vi "Verificador_leitura_de_forma.vi"() -> ()   [LabVIEW 2017]
uses:
  <vilib>/userdefined/High Color/IMAQdx.ctl
  <vilib>/vision/driver/IMAQdx.llb/IMAQdx Acquisition Mode.ctl
  <vilib>/vision/driver/IMAQdx.llb/IMAQdx Buffer Number Mode.ctl
  <vilib>/vision/Classification.llb/IMAQ Classifier Read Options.ctl
  <vilib>/vision/driver/NI_Vision_Acquisition_Software.lvlib
  <vilib>/vision/NI_Vision_Development_Module.lvlib
panel:
  out "Forma 2":string
  out "Imagem Original 2":T1(plugin-control)
  out "Session Out":T2
  out "error out":errorcluster
  out "Forma":string
  out "Points":cluster{"X":dbl, "Y":dbl}[](array[cluster])
  in  "error in":errorcluster
  out "Stop 3":bool
  out "lista":enum16{"normal", "detectou", "parou"}(ring)=enum."detectou"
  in  "enum":enum16{"normal", "detectou", "parou"}(ring)=enum."detectou"
  in  "Stop Button":bool
  in  "largura_y":sgl=30.0
  in  "largura_x":sgl=30.0
  in  "ofset y":sgl
  in  "ofset x":sgl
  in  "Tab Control":T3(tab)
  in  "Stop 2":bool
  in  "Stop 1":bool
  out "Imagem Original":T1(plugin-control)
  in  "Câmera":T2="cam1"
  # "0"
  # "-250"
  # "400"
  # "80"
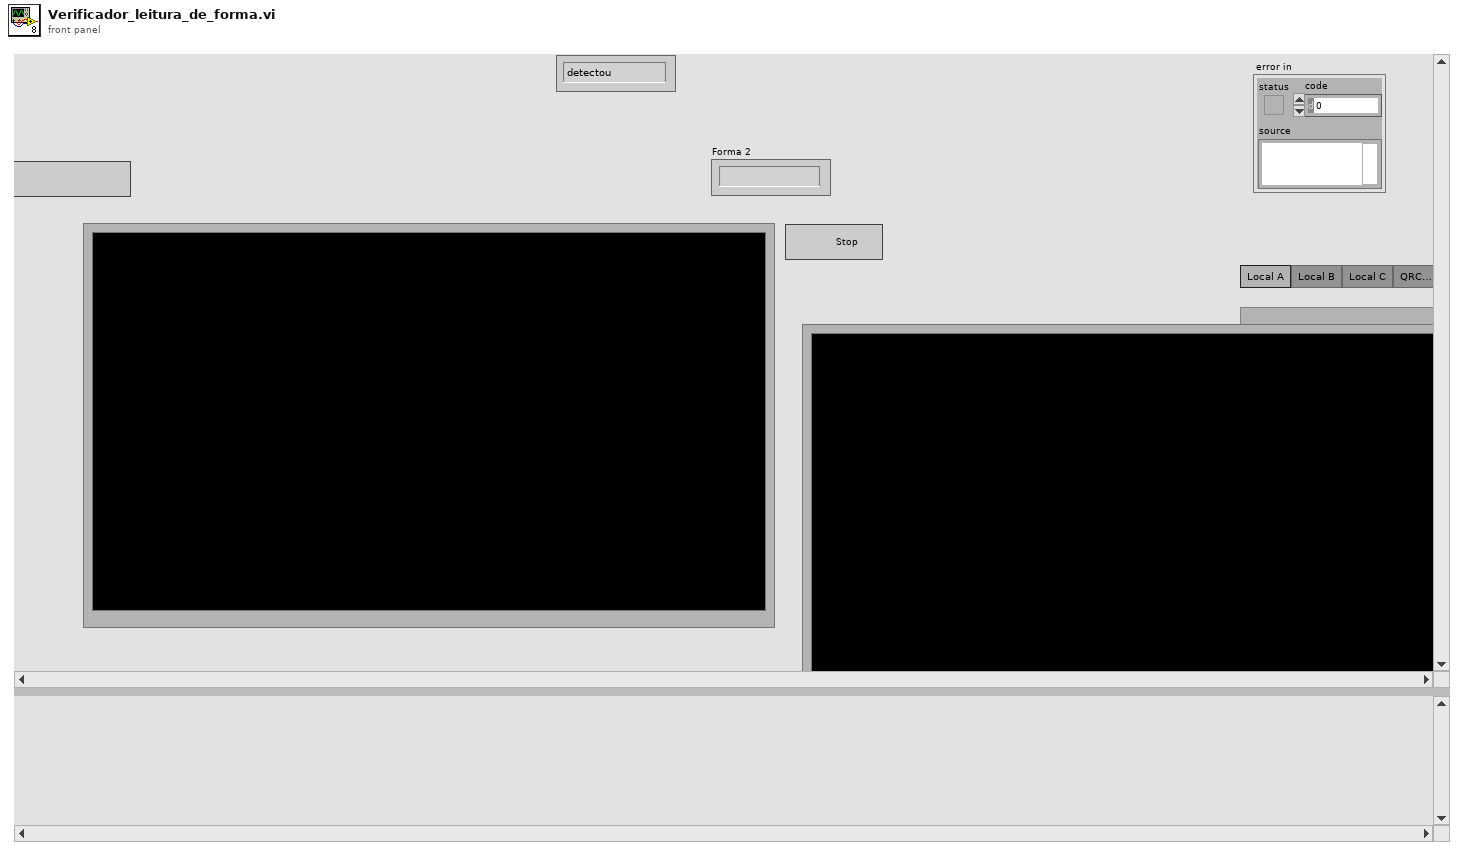
[diagram p1: front panel]
types:
  T1 = typedef "IMAQ Image.ctl" = refnum<image>
  T2 = typedef "IMAQdx.ctl" = refnum<k21>
  T3 = enum32{"Local A", "Local B", "Local C", "QRCode"}
  T4 = typedef "NI_Vision_Acquisition_Software.lvlib/IMAQdx Acquisition Mode.ctl" = enum32{"One Shot", "Continuous"}
  T5 = typedef "NI_Vision_Acquisition_Software.lvlib/IMAQdx Buffer Number Mode.ctl" = enum32{"Next", "Last", "Buffer Number", "Every", "Last New"}
  T6 = cluster{"Global Rectangle":i32[], "Contours":cluster{"Contour Type":u32, "ROI Type":u32, "Points":i32[]}[]}
  T7 = enum32{"AutoM", "Close", "Dilate", "Erode", "Gradient", "Gradient out", "Gradient in", "Hit miss", "Open", "PClose", "POpen", "Thick", "Thin"}
  T8 = typedef "ROI Descriptor" = cluster{"Global Rectangle":i32[], "Contours":cluster{"ID":enum32{"External", "Internal"}, "Type":u32, "Coordinates":i32[]}[]}
  T9 = typedef "IMAQ Classifier Read Options.ctl" = i32
  T10 = typedef "IMAQ Classifier Session.ctl" = refnum<k1>
  T11 = cluster{"Contour Type":u32, "ROI Type":u32, "Points":i32[]}[]
  T12 = cluster{"Contour Type":u32, "ROI Type":u32, "Points":i32[]}
  T13 = typedef "Image Type" = u32
  T14 = typedef "IMAQ ExtractCurvesCurve.ctl" = cluster{"Points":cluster{"X":dbl, "Y":dbl}[], "Closed?":bool, "Curve Length":dbl, "Min Edge Strength":dbl, "Max Edge Strength":dbl, "Average Edge Strength":dbl}
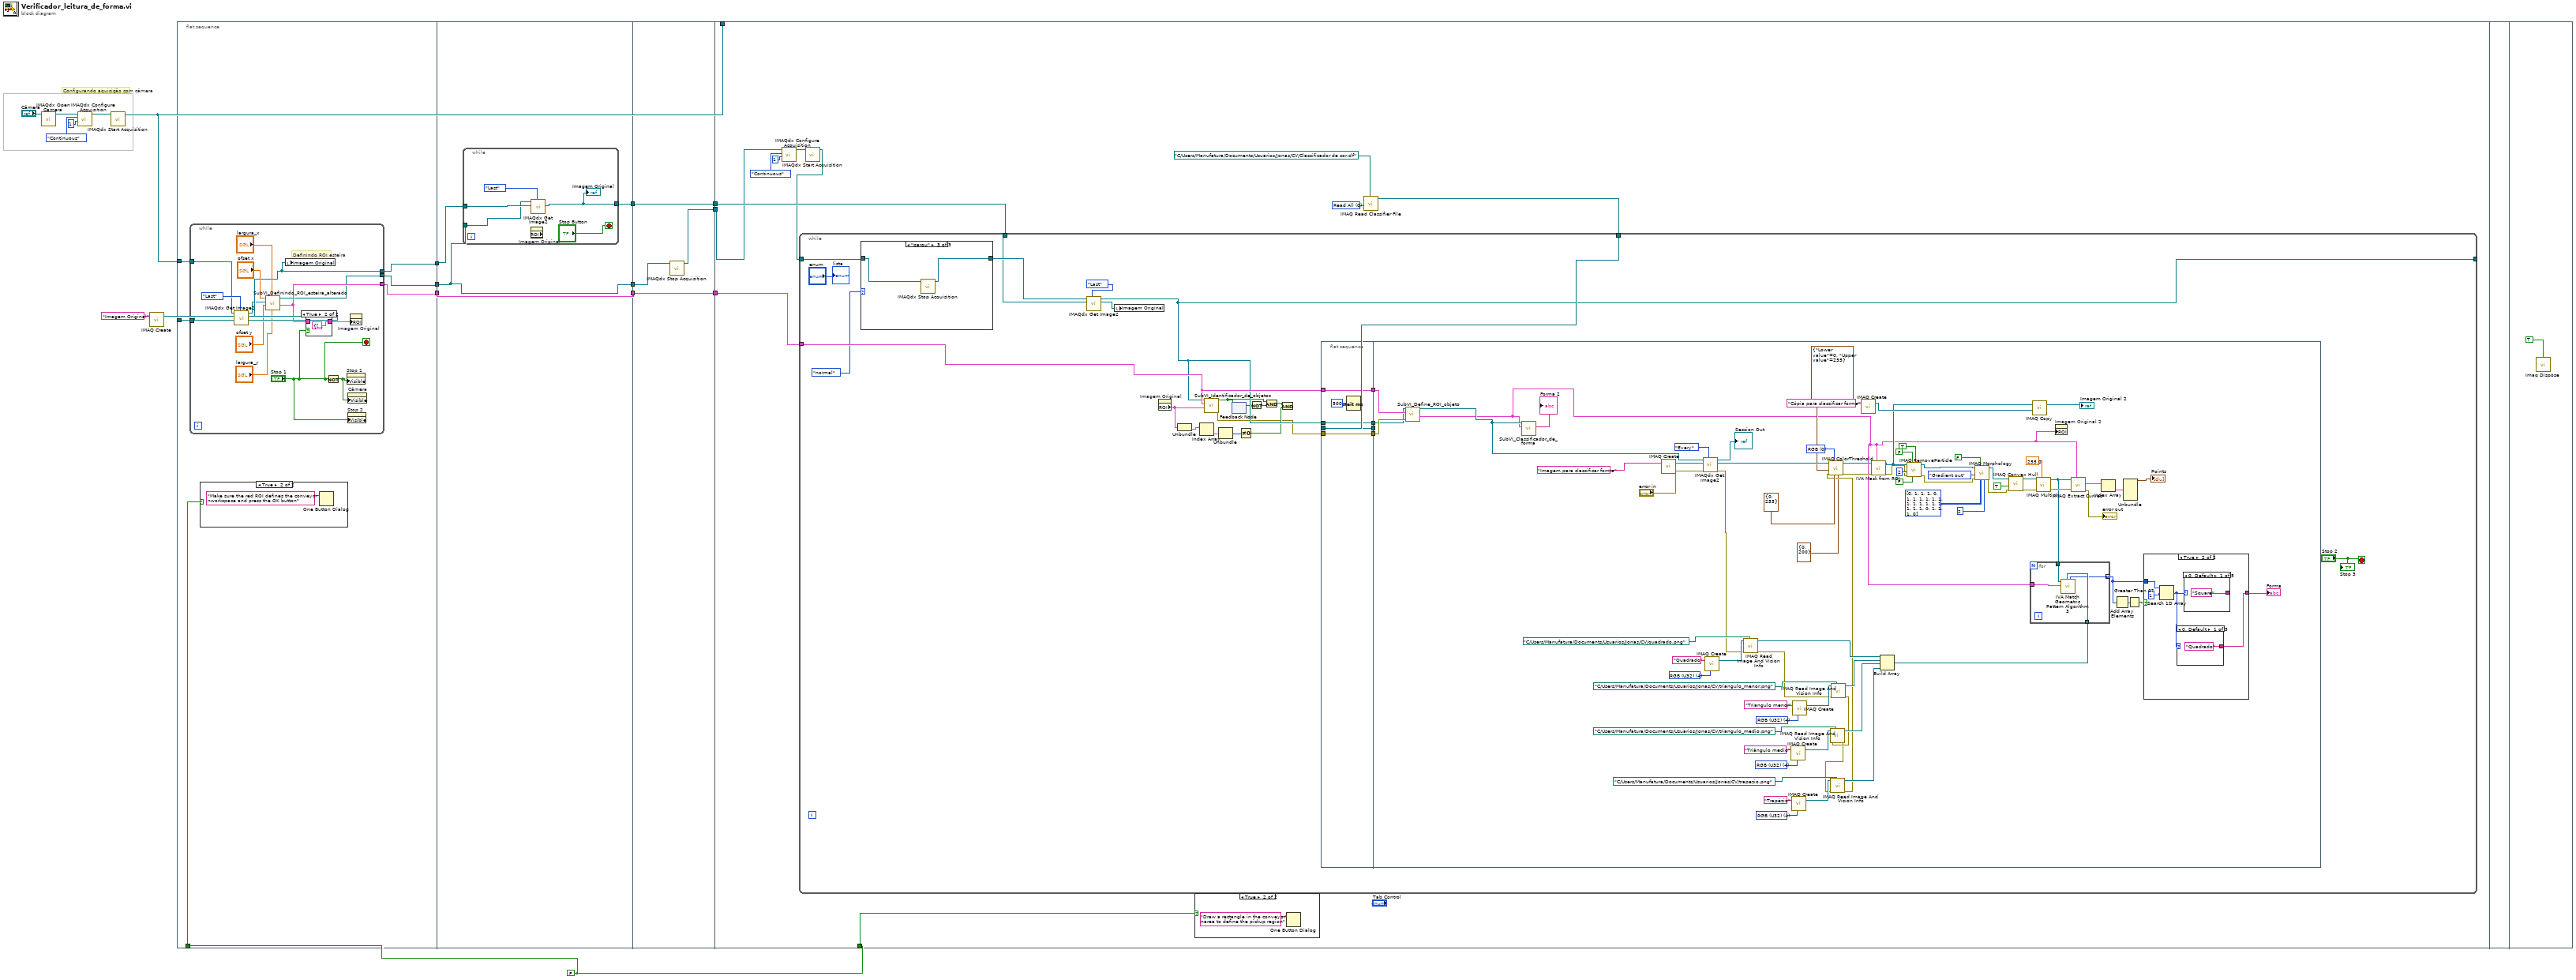
[diagram p0: block diagram]
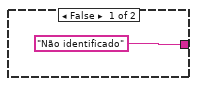
[diagram p4: hidden frame]
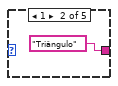
[diagram p5: hidden frame]
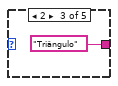
[diagram p6: hidden frame]
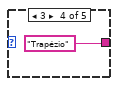
[diagram p7: hidden frame]
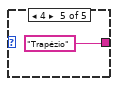
[diagram p8: hidden frame]
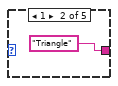
[diagram p9: hidden frame]
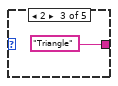
[diagram p10: hidden frame]
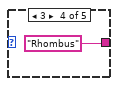
[diagram p11: hidden frame]
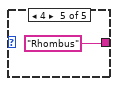
[diagram p12: hidden frame]
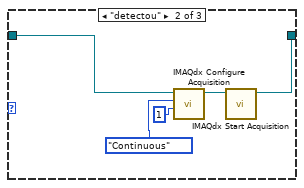
[diagram p14: hidden frame]
diagram:
  w11 = FALSE
  # "Configurando aquisição com câmera"
  n1 = call <vilib>:"IMAQdx Open Camera.vi"("Session In"="Câmera") -> ("Session Out"=w18:T2)  [unwired: 9 in, 1 out]
  n2 = call <vilib>:"IMAQdx Configure Acquisition.vi"("Number of Buffers"=u32 1, "Continuous?"=IMAQdx_Acquisition_Mode."Continuous", "Session In"=w18) -> ("Session Out"=w17:T2)  [unwired: 7 in, 1 out]
  n3 = call <vilib>:"IMAQdx Start Acquisition.vi"("Session In"=w17) -> ("Session Out"=w2:T2)  [unwired: 9 in, 1 out]
  n4 = call "IMAQ Create"("Image Name"="Imagem Original") -> ("New Image"=w12:T1)  [unwired: 4 in, 1 out]
  n5 = flat-sequence {
    tunnel: w2 -> [w24]
    tunnel: w12 -> [w23]
    tunnel: [w22] -> w10
    tunnel: [w21] -> w9
    tunnel: [w20] -> w8
    tunnel: w11 -> [w19]
    tunnel: w10 -> [w42]
    tunnel: [w42] -> w7
    tunnel: w9 -> [w45]
    tunnel: [w45] -> w6
    tunnel: w8 -> [w43]
    tunnel: [w44] -> w3
    tunnel: w7 -> [w53]
    tunnel: w6 -> [w54]
    tunnel: [w54] -> w5
    tunnel: [w52] -> w4
    tunnel: w3 -> [w52]
    tunnel: [w51] -> w1
    tunnel: w5 -> [w61]
    tunnel: w11 -> [w65]
    tunnel: w4 -> [w60]
    tunnel: w2 -> [_]
    tunnel: w1 -> [w56]
    frame #0 {
      n6 = while {
        tunnel: w24 -> [w38]
        tunnel: w23 -> [w37]
        tunnel: [w26] -> w22
        tunnel: [w27] -> w21
        tunnel: [w35] -> w20
        stop <- "Stop 1" stop-if-true
        # "Definindo ROI esteira"
        n7 = call <vilib>:"IMAQdx Get Image2.vi"("Buffer Number Mode (Next)"=IMAQdx_Buffer_Number_Mode."Last", "Image In"=w37, "Session In"=w38) -> ("Image Out"=w35:T1, "Session Out"=w28:T2)  [unwired: 5 in, 2 out]
        n8 = call "SubVI_Definindo_ROI_esteira_alterado.vi"("largura_y"="largura_y", "largura_x"="largura_x", "ofset y"="ofset y", "Session in"=w28, "ofset x"="ofset x") -> ("ROI Descriptor"=w27:T8, "Session Out"=w26:T2)  [unwired: 4 in, 1 out]
        n9 = local write "Imagem Original"(w35) -> ()
        n10 = case shown="True" "Stop 1" {
          tunnel: w27 -> [w40 _]
          tunnel: [w40 T6 {"Global Rectangle"=[0, 0, 1, 1], "Contours"=[{"Contour Type"=0, "ROI Type"=1, "Points"=[0, 0]}]} ("ROI")] -> w36
          frame False {
          }
          frame True {
          }
        }
        n11 = Not(x="Stop 1") -> (.not. x?=w34:bool)
        n12 = property on="Stop 1" class="Bool"("Visible"=w34) -> ()  [unwired: 2 in, 2 out]
        n13 = property on="Stop 2" class="Bool"("Visible"="Stop 1") -> ()  [unwired: 2 in, 2 out]
        n14 = property on="Câmera" class="IMAQdx (strict)"("Visible"=w34) -> ()  [unwired: 2 in, 2 out]
        n15 = property on="Imagem Original" class="ImageControl"("ROI"=w36) -> ()  [unwired: 2 in, 2 out]
      }
      n16 = case shown="True" w19 {
        frame False {
        }
        frame True {
          n17 = One Button Dialog(message="Make sure the red ROI defines the conveyor \nworkspace and press the OK button") -> ()  [unwired: 1 in, 1 out]
        }
      }
    }
    frame #1 {
      n18 = while {
        tunnel: w43 -> [w49]
        tunnel: w42 -> [w46]
        tunnel: [w47] -> w44
        stop <- "Stop Button" stop-if-true
        n19 = property on="Imagem Original" class="ImageControl" props=["ROI"]() -> ()  [unwired: 2 in, 3 out]
        n20 = call <vilib>:"IMAQdx Get Image2.vi"("Buffer Number Mode (Next)"=IMAQdx_Buffer_Number_Mode."Last", "Image In"=w49, "Session In"=w46) -> ("Image Out"=w47:T1)  [unwired: 5 in, 3 out]
        "Imagem Original" <- w47
      }
    }
    frame #2 {
      n21 = call <vilib>:"IMAQdx Stop Acquisition.vi"("Session In"=w53) -> ("Session Out"=w51:T2)  [unwired: 9 in, 1 out]
    }
    frame #3 {
      w64 = T9 0 items=["Read All", "Add Samples, Do Not Change Options", "Read Options, Do Not Add Samples"] ("Read Options")
      n22 = call <vilib>:"IMAQdx Configure Acquisition.vi"("Number of Buffers"=u32 1, "Continuous?"=IMAQdx_Acquisition_Mode."Continuous", "Session In"=w56) -> ("Session Out"=w57:T2)  [unwired: 7 in, 1 out]
      n23 = call <vilib>:"IMAQdx Start Acquisition.vi"("Session In"=w57) -> ("Session Out"=w55:T2)  [unwired: 9 in, 1 out]
      n24 = case shown="True" w65 {
        frame False {
        }
        frame True {
          n25 = One Button Dialog(message="Draw a rectangle in the conveyor\narea to define the pickup region") -> ()  [unwired: 1 in, 1 out]
        }
      }
      n26 = call "IMAQ Read Classifier File"("File Path"=path "C:/Users/Manufatura/Documents/Usuarios/Jonas/CV/Classificador de cor.clf", "Read Options"=w64) -> ("Classifier Session"=w63:T10)  [unwired: 2 in, 7 out]
      n27 = while {
        tunnel: w61 -> [w89]
        tunnel: w63 -> [w90]
        tunnel: w60 -> [w87]
        tunnel: w55 -> [w85]
        tunnel: [w86] -> _
        stop <- "Stop 2" stop-if-true
        n28 = case shown="\"parou\"" enum16{"normal", "detectou", "parou"}."normal" {
          tunnel: [w190 w191 w196] -> w88
          tunnel: w85 -> [w190 w192 w197]
          frame "normal", Default {
          }
          frame "detectou" {
            n29 = call <vilib>:"IMAQdx Configure Acquisition.vi"("Number of Buffers"=u32 1, "Continuous?"=IMAQdx_Acquisition_Mode."Continuous", "Session In"=w192) -> ("Session Out"=w193:T2)  [unwired: 7 in, 1 out]
            n30 = call <vilib>:"IMAQdx Start Acquisition.vi"("Session In"=w193) -> ("Session Out"=w191:T2)  [unwired: 9 in, 1 out]
          }
          frame "parou" {
            n31 = call <vilib>:"IMAQdx Stop Acquisition.vi"("Session In"=w197) -> ("Session Out"=w196:T2)  [unwired: 9 in, 1 out]
          }
        }
        n32 = call <vilib>:"IMAQdx Get Image2.vi"("Buffer Number Mode (Next)"=IMAQdx_Buffer_Number_Mode."Last", "Image In"=w87, "Session In"=w88) -> ("Image Out"=w66:T1, "Session Out"=w86:T2)  [unwired: 5 in, 2 out]
        n33 = local write "Imagem Original"(w66) -> ()
        n34 = property on="Imagem Original" class="ImageControl"() -> ("ROI"=w77:T6)  [unwired: 2 in, 2 out]
        n35 = Unbundle(w77) -> ("Contours"=w76:T11)  [unwired: 1 out]
        n36 = Index Array(array=w76) -> (element=w75:T12)  [unwired: 1 in]
        n37 = call "SubVI_Identificador_de_objetos.vi"("ROI Detecção"=w77, "ROI Esteira"=w89, "Session In"=w86) -> ("error out"=w72:errorcluster, "Objeto Identificado"=w70:bool)  [unwired: 7 in]
        n38 = Unbundle(w75) -> ("ROI Type"=w74:u32)  [unwired: 2 out]
        n39 = feedback #1() -> (w69:bool)  [unwired: 1 in]
        n40 = feedback-in #1(w70) -> ()
        n41 = Not Equal To 0?(x=w74) -> (x != 0?=w73:bool)
        n42 = Not(x=w69) -> (.not. x?=w68:bool)
        n43 = And(x=w70, y=w68) -> (x .and. y?=w71:bool)
        n44 = And(x=w71, y=w73) -> ()  [unwired: 1 out]
        n45 = flat-sequence {
          tunnel: [w95] -> w81
          tunnel: [w94] -> w80
          tunnel: [w93] -> w79
          tunnel: [w92] -> w78
          tunnel: w90 -> [w95]
          tunnel: w72 -> [w94]
          tunnel: w86 -> [w93]
          tunnel: w89 -> [w92]
          tunnel: w81 -> [_]
          tunnel: w80 -> [w169]
          tunnel: w79 -> [w168]
          tunnel: w78 -> [w170]
          frame #0 {
            n46 = Wait (ms)(milliseconds to wait=u32 500) -> ()  [unwired: 1 out]
          }
          frame #1 {
            w128 = T13 4 items=["Grayscale (U8)", "Grayscale (I16)", "Grayscale (SGL)", "Complex (CSG)", "RGB (U32)", "HSL (U32)", "RGB (U64)", "Grayscale (U16)"] ("Image Type")
            w133 = T13 4 items=["Grayscale (U8)", "Grayscale (I16)", "Grayscale (SGL)", "Complex (CSG)", "RGB (U32)", "HSL (U32)", "RGB (U64)", "Grayscale (U16)"] ("Image Type")
            w136 = T13 4 items=["Grayscale (U8)", "Grayscale (I16)", "Grayscale (SGL)", "Complex (CSG)", "RGB (U32)", "HSL (U32)", "RGB (U64)", "Grayscale (U16)"] ("Image Type")
            w141 = T13 4 items=["Grayscale (U8)", "Grayscale (I16)", "Grayscale (SGL)", "Complex (CSG)", "RGB (U32)", "HSL (U32)", "RGB (U64)", "Grayscale (U16)"] ("Image Type")
            w162 = u16 0 items=["RGB", "HSL", "HSV", "HSI"] ("Color Mode")
            n47 = call "SubVI_Define_ROI_objeto.vi"("error in (no error)"=w169, "ROI Esteira"=w170, "Session In"=w168) -> ("ROI Objeto"=w97:T8, "Session Out"=w98:T2)  [unwired: 5 in, 2 out]
            n48 = call "SubVI_Classificador_de_forma.vi"("ROI Objeto"=w97, "Session In"=w98) -> ("Forma"=→"Forma 2":string)  [unwired: 6 in, 3 out]
            n49 = call "IMAQ Create"("Image Name"="Imagem para classificar forma") -> ("New Image"=w165:T1)  [unwired: 4 in, 1 out]
            n50 = call <vilib>:"IMAQdx Get Image2.vi"("Buffer Number Mode (Next)"=IMAQdx_Buffer_Number_Mode."Every", "error in"="error in", "Image In"=w165, "Session In"=w98) -> ("error out"=w111:errorcluster, "Image Out"=w163:T1, "Session Out"=→"Session Out":T2)  [unwired: 4 in, 1 out]
            n51 = call "IMAQ Create"("Image Name"="Quadrado", "Image Type"=w141) -> ("New Image"=w140:T1)  [unwired: 3 in, 1 out]
            n52 = call "IMAQ Read Image And Vision Info"("File Path"=path "C:/Users/Manufatura/Documents/Usuarios/Jonas/CV/quadrado.png" ("Template File Path"), "error in (no error)"=w111, "Image"=w140) -> ("error out"=w110:errorcluster, "Image Out"=w126:T1)  [unwired: 1 in, 6 out]
            n53 = call "IMAQ Create"("Image Name"="Triângulo medio", "Image Type"=w136) -> ("New Image"=w137:T1)  [unwired: 3 in, 1 out]
            n54 = call "IMAQ Create"("Image Name"="Trapézio", "Image Type"=w133) -> ("New Image"=w132:T1)  [unwired: 3 in, 1 out]
            n55 = call "IMAQ Create"("Image Name"="Triangulo menor", "Image Type"=w128) -> ("New Image"=w129:T1)  [unwired: 3 in, 1 out]
            n56 = call "IMAQ Read Image And Vision Info"("File Path"=path "C:/Users/Manufatura/Documents/Usuarios/Jonas/CV/triangulo_menor.png" ("Template File Path"), "error in (no error)"=w110, "Image"=w129) -> ("error out"=w109:errorcluster, "Image Out"=w125:T1)  [unwired: 1 in, 6 out]
            n57 = call "IMAQ Read Image And Vision Info"("File Path"=path "C:/Users/Manufatura/Documents/Usuarios/Jonas/CV/triangulo_medio.png" ("Template File Path"), "error in (no error)"=w109, "Image"=w137) -> ("error out"=w108:errorcluster, "Image Out"=w124:T1)  [unwired: 1 in, 6 out]
            n58 = call "IMAQ Read Image And Vision Info"("File Path"=path "C:/Users/Manufatura/Documents/Usuarios/Jonas/CV/trapezio.png" ("Template File Path"), "error in (no error)"=w108, "Image"=w132) -> ("error out"=w107:errorcluster, "Image Out"=w123:T1)  [unwired: 1 in, 6 out]
            n59 = call "IMAQ ColorThreshold"("Blue or Luma or Val or Inten Range"=cluster{"Lower value":i32, "Upper value":i32} {"Lower value"=0, "Upper value"=200}, "Green or Sat Range"=cluster{"Lower value":i32, "Upper value":i32} {"Lower value"=0, "Upper value"=255}, "Color Mode"=w162, "error in (no error)"=w107, "Red or Hue Range"=cluster{"Lower value":i32, "Upper value":i32} {"Lower value"=0, "Upper value"=255}, "Image Src"=w163) -> ("error out"=w120:errorcluster, "Image Dst Out"=w159:T1)  [unwired: 2 in, 2 out]
            n60 = call "IMAQ Create"("Image Name"="Cópia para classificar forma") -> ("New Image"=w101:T1)  [unwired: 4 in, 1 out]
            n61 = call <vilib>:"IVA Mask from ROI.vi"("ROI Descriptor"=w97, "error in (no error)"=w120, "Image Src"=w159) -> ("error out"=w119:errorcluster, "Image Out"=w100:T1)  [unwired: 2 in, 5 out]
            n62 = Build Array(w126, w125, w124, w123) -> (w122:T1[])
            n63 = call "IMAQ RemoveParticle"("Connectivity 4/8 (8)"=TRUE, "Low Pass/High Pass (Low)"=FALSE, "Square/Hexa (Square)"=FALSE, "error in (no error)"=w119, "Number of Erosion"=2, "Image Src"=w100) -> ("error out"=w118:errorcluster, "Image Dst Out"=w152:T1)  [unwired: 1 in, 3 out]
            n64 = call "IMAQ Morphology"("Number of iterations (1)"=2, "Structuring Element"=i32[][] [[0, 1, 1, 1, 0], [1, 1, 1, 1, 1], [1, 1, 1, 1, 1], [1, 1, 1, 1, 1], [0, 1, 1, 1, 0]], "Square/Hexa (Square)"=FALSE, "error in (no error)"=w118, "Operation"=T7."Gradient out", "Image Src"=w152) -> ("error out"=w117:errorcluster, "Image Dst Out"=w148:T1)  [unwired: 1 in, 3 out]
            n65 = call "IMAQ Convex Hull"("error in (no error)"=w117, "Connectivity 4/8 (8)"=TRUE, "Image Src"=w148) -> ("error out"=w116:errorcluster, "Image Dst Out"=w146:T1)  [unwired: 1 in, 6 out]
            n66 = call "IMAQ Copy"("Image Dst"=w101, "Image Src"=w100) -> ("Image Dst Out"=→"Imagem Original 2":T1)  [unwired: 4 in, 1 out]
            n67 = call "IMAQ Multiply"("Image Src A"=w146, "Constant"=255.0, "error in (no error)"=w116) -> ("Image Dst Out"=w104:T1, "error out"=w112:errorcluster)  [unwired: 4 in]
            n68 = for {
              tunnel: w122 -> [w187] mode=indexing
              tunnel: w97 -> [w189]
              tunnel: w104 -> [w188]
              tunnel: [w186] -> w114 mode=indexing
              n69 = call <vilib>:"IVA Match Geometric Pattern Algorithm 3.vi"("Template"=w187, "ROI Descriptor"=w189, "Image"=w188) -> ("Number of Matches"=w186:i32)  [unwired: 2 in, 6 out]
            }
            n70 = property on="Imagem Original 2" class="ImageControl"("ROI"=w97) -> ()  [unwired: 2 in, 2 out]
            n71 = call "IMAQ Extract Curves"("ROI Descriptor"=w97, "error in (no error)"=w112, "Image"=w104) -> ("error out"=→"error out":errorcluster, "Curves"=w144:T14[])  [unwired: 6 in, 1 out]
            n72 = Index Array(array=w144) -> (element=w145:T14)  [unwired: 1 in]
            n73 = Add Array Elements(numeric array=w114) -> (sum=w115:i32)
            n74 = Unbundle(w145) -> ("Points"=→"Points":cluster{"X":dbl, "Y":dbl}[])  [unwired: 5 out]
            n75 = Greater Than 0?(x=w115) -> (x > 0?=w113:bool)
            n76 = case shown="True" w113 {
              tunnel: w114 -> [_ w175]
              tunnel: ["Não identificado" w172] -> w121
              frame False {
              }
              frame True {
                n77 = Search 1D Array(1D array=w175, element=1) -> (index of element=w173:i32)  [unwired: 1 in]
                n78 = case shown="0, Default" w173 {
                  tunnel: ["Quadrado" "Triângulo" "Triângulo" "Trapézio" "Trapézio"] -> w172
                  frame 0, Default {
                  }
                  frame 1 {
                  }
                  frame 2 {
                  }
                  frame 3 {
                  }
                  frame 4 {
                  }
                }
                n79 = case shown="0, Default" w173 {
                  tunnel: ["Square" "Triangle" "Triangle" "Rhombus" "Rhombus"] -> _
                  frame 0, Default {
                  }
                  frame 1 {
                  }
                  frame 2 {
                  }
                  frame 3 {
                  }
                  frame 4 {
                  }
                }
              }
            }
            "Forma" <- w121
          }
        }
        "lista" <- "enum"
        "Stop 3" <- "Stop 2"
      }
    }
    frame #4 {
    }
    frame #5 {
      n80 = call "Imaq Dispose"("All Images? (No)"=TRUE) -> ()  [unwired: 5 in, 1 out]
    }
  }
